vi "Calibrate_Short.vi"(8 "error in":errorcluster, 9 "Keystate":string, 10 "Stop Test":bool=TRUE, 11 "Calibration Test":bool=TRUE) -> (0 "error out":errorcluster, 5 "Calibration Short Successful":bool)   [LabVIEW 2020]
uses:
  <vilib>/Instr/_visa.llb/GPIB Status Boolean Array.ctl
  <vilib>/Utility/error.llb/DialogType.ctl
panel:
  out "ibsta":T1
  out "message":string=" INSTRUCTIONS:\r\rNormal Use:  When using subVIs that incorporate the error in/error out (or error I/O) structure, place this handler where you want to inform the user of an error, typically at the end of the I/O data path, as the last action of the program.  If the error in error? is ERROR, the handler creates a message describing the error and its source.  If the type of dialog = 1 (default), the message is displayed to the user, who can only acknowedge it.  If the type = 2, the user can acknowledge the message or abort execution; aborting a program with active I/O is not recommended.  If the type = 0, no message is displayed; this is used to process the error programmatically, and the error out cluster elements are wired to individual terminals for that reason.  \r\rOther Use:\n\r\nlocal testing.  To test the error code of a subVI or function that does not have the error I/O structure, you can wire its error code and a source string to the local error code and error source inputs.  If error in error? indicates no error and error code is not equal to 0, the local code and source are substituted for the error in values, and error? is set TRUE (ERROR)."
  out "Test Count":i32
  out "Failed Test Count":i32
  out "serial poll byte (Test 2)":i16
  out "serial poll byte (Test 1)":i16
  in  "Test Failed":bool=TRUE
  in  "Cal_Step_Delay":u16
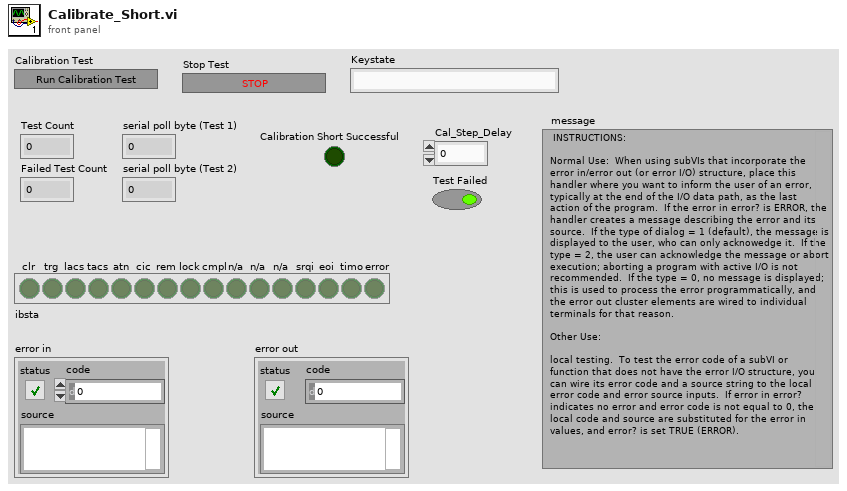
[diagram p1: front panel]
types:
  T1 = typedef "GPIB Status Boolean Array.ctl" = bool[]
  T2 = typedef "DialogType.ctl" = u16
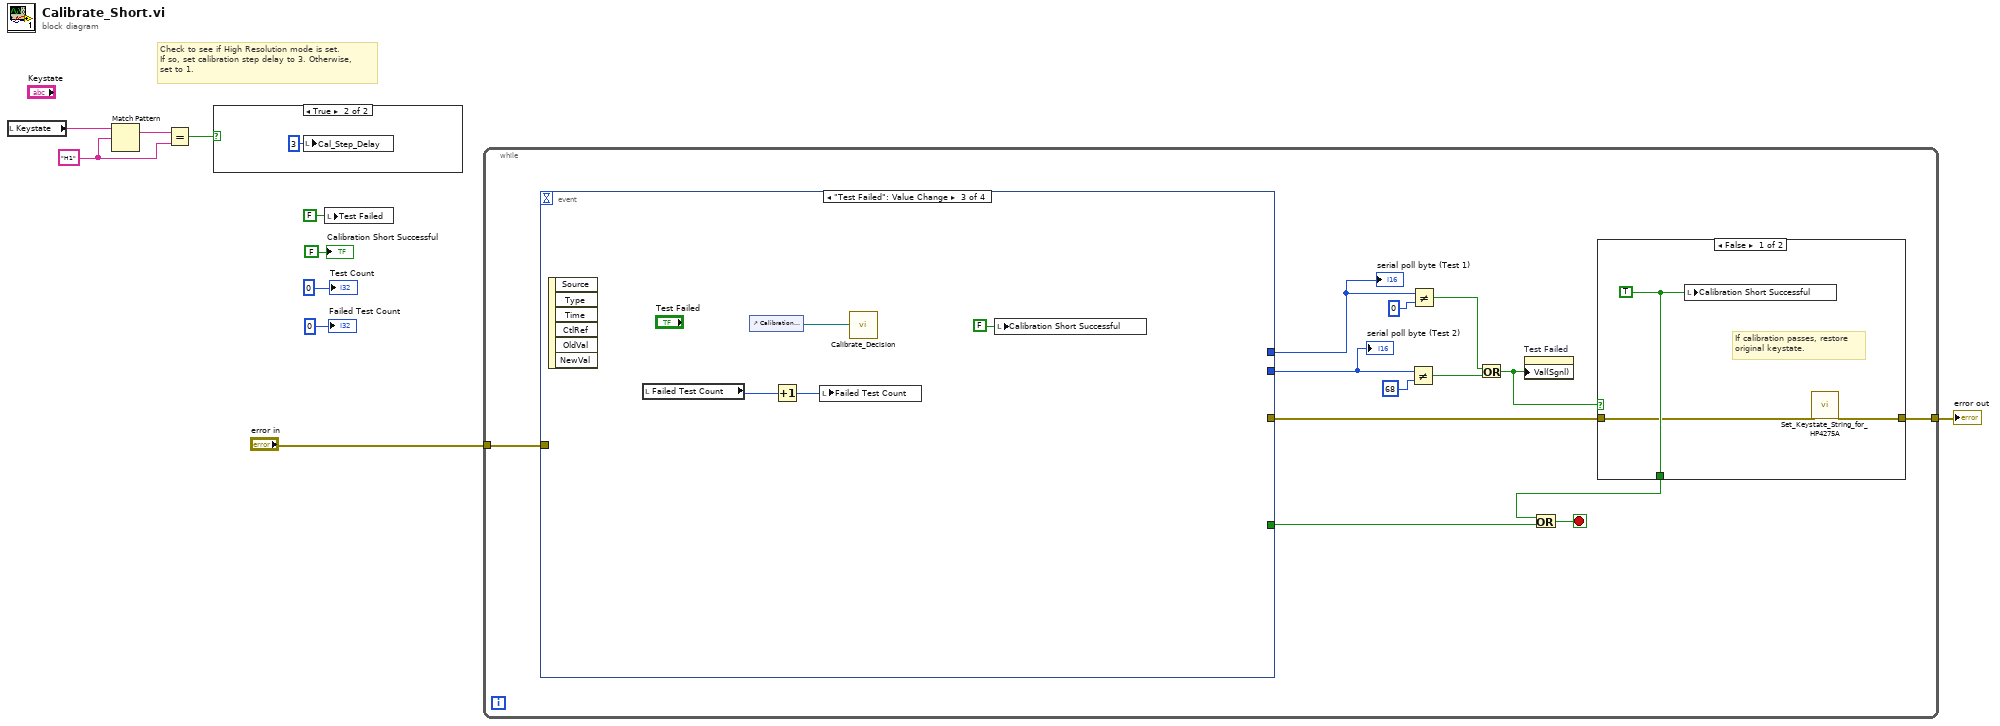
[diagram p0: block diagram]
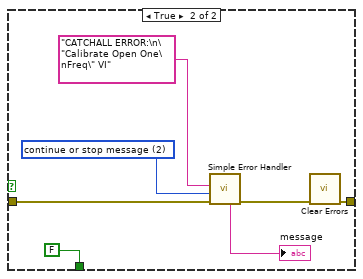
[diagram p2: hidden frame]
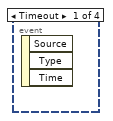
[diagram p3: hidden frame]
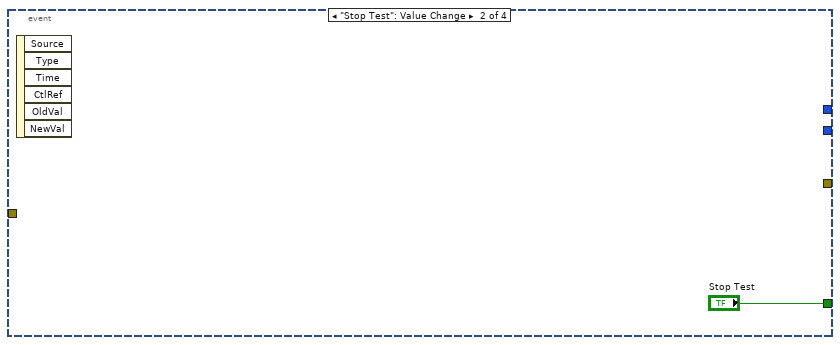
[diagram p4: hidden frame]
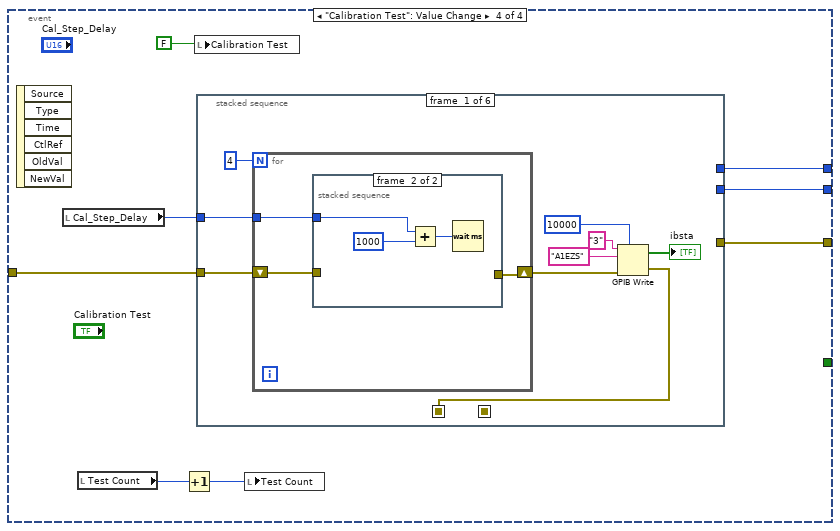
[diagram p5: hidden frame]
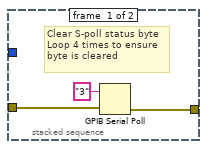
[diagram p6: hidden frame]
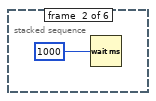
[diagram p7: hidden frame]
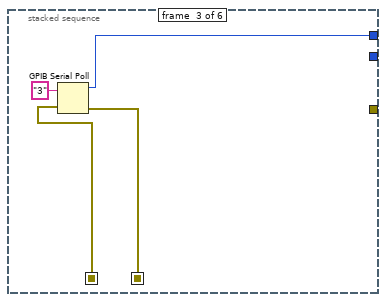
[diagram p8: hidden frame]
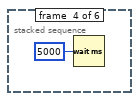
[diagram p9: hidden frame]
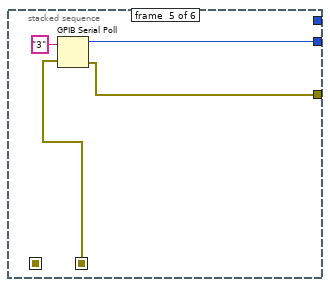
[diagram p10: hidden frame]
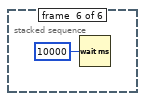
[diagram p11: hidden frame]
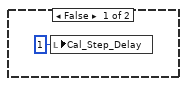
[diagram p12: hidden frame]
diagram:
  w10 = "H1" ("regular expression")
  # "Check to see if High Resolution mode is set.\nIf so, set calibration step delay to 3. Otherwise,\nset to 1."
  n1 = local read "Keystate"() -> (w6:string)
  n2 = Match Pattern(string=w6, regular expression=w10) -> (match substring=w9:string)  [unwired: 1 in, 3 out]
  n3 = Equal?(x=w9, y=w10) -> (x = y?=w8:bool)
  n4 = case shown="True" w8 {
    frame False {
      n5 = local write "Cal_Step_Delay"(u16 1 ("CalStepDelay")) -> ()
    }
    frame True {
      n6 = local write "Cal_Step_Delay"(u16 3 ("CalStepDelay")) -> ()
    }
  }
  n7 = local write "Test Failed"(FALSE ("Test Failed")) -> ()
  n8 = while {
    tunnel: "error in" -> [w25]
    tunnel: [w20] -> w7
    stop <- w22 stop-if-true
    n9 = event shown="[2] \"Test Failed\": Value Change" {
      selector: _ -> [_ _ _ _]
      dyn-events: _ -> [_ _ _ _]
      timeout: _ -> [_ _ _ _]
      tunnel: w25 -> [_ _ _ w48]
      tunnel: [_ _ _ w46] -> w21
      tunnel: [_ "Stop Test" _ _] -> w23
      tunnel: [_ _ _ w42] -> w17
      tunnel: [_ _ _ w41] -> w14
      event Timeout {
        n10 = event-data() -> ()  [unwired: 1 in, 3 out]
      }
      event "Stop Test": Value Change {
        n11 = event-data() -> ()  [unwired: 1 in, 6 out]
      }
      event "Test Failed": Value Change {
        n12 = event-data() -> ()  [unwired: 1 in, 6 out]
        n13 = local read "Failed Test Count"() -> (w40:i32)
        n14 = control-ref of="Calibration Test"() -> (w38:refnum<vi>)
        n15 = Increment(x=w40) -> (x+1=w39:i32)
        n16 = local write "Failed Test Count"(w39) -> ()
        n17 = call "Calibrate_Decision.vi"("reference"=w38) -> ()  [unwired: 11 in]
        n18 = local write "Calibration Short Successful"(FALSE ("Calibration Short Successful")) -> ()
      }
      event "Calibration Test": Value Change {
        n19 = event-data() -> ()  [unwired: 1 in, 6 out]
        n20 = local read "Cal_Step_Delay"() -> (w47:u16)
        n21 = local read "Test Count"() -> (w44:i32)
        n22 = Increment(x=w44) -> (x+1=w43:i32)
        n23 = local write "Calibration Test"(FALSE ("Calibration Test")) -> ()
        n24 = stacked-sequence {
          seq-local: [w49 _ _ _ _ _] -> [_ _ w70 _ _ _]
          seq-local: [_ _ w69 _ _ _] -> [_ _ _ _ w75 _]
          tunnel: w48 -> [w57 _ _ _ _ _]
          tunnel: w47 -> [w56 _ _ _ _ _]
          tunnel: [_ _ _ _ w74 _] -> w46
          tunnel: [_ _ w68 _ _ _] -> w42
          tunnel: [_ _ _ _ w73 _] -> w41
          frame #0 {
            n25 = for {
              N: 4 -> [_]
              tunnel: w56 -> [w59]
              shift-right: [w58] -> w50
              shift-left: w57 -> [w60]
              n26 = stacked-sequence {
                tunnel: w60 -> [w62 _]
                tunnel: w59 -> [_ w65]
                tunnel: [w61 _] -> w58
                frame #0 {
                  # "Clear S-poll status byte\nLoop 4 times to ensure\nbyte is cleared"
                  n27 = GPIB Serial Poll(0:"3" ("address string"), 1:w62) -> (4:w61:errorcluster)  [unwired: 2 out]
                }
                frame #1 {
                  n28 = Add(x=w65, y=u32 1000 ("milliseconds to wait")) -> (x+y=w64:u32)
                  n29 = Wait (ms)(milliseconds to wait=w64) -> ()  [unwired: 1 out]
                }
              }
            }
            n30 = GPIB Write(0:"3" ("address string"), 1:"A1EZS" ("data"), 3:w50, 4:10000 ("timeout ms (488.2 global)")) -> (5:→"ibsta":bool[], 6:w49:errorcluster)  [unwired: 1 in]
          }
          frame #1 {
            n31 = Wait (ms)(milliseconds to wait=u32 1000) -> ()  [unwired: 1 out]
          }
          frame #2 {
            n32 = GPIB Serial Poll(0:"3" ("address string"), 1:w70) -> (2:w68:i16, 4:w69:errorcluster)  [unwired: 1 out]
          }
          frame #3 {
            n33 = Wait (ms)(milliseconds to wait=u32 5000) -> ()  [unwired: 1 out]
          }
          frame #4 {
            n34 = GPIB Serial Poll(0:"3" ("address string"), 1:w75) -> (2:w73:i16, 4:w74:errorcluster)  [unwired: 1 out]
          }
          frame #5 {
            n35 = Wait (ms)(milliseconds to wait=u32 10000) -> ()  [unwired: 1 out]
          }
        }
        n36 = local write "Test Count"(w43) -> ()
      }
    }
    "serial poll byte (Test 1)" <- w17
    "serial poll byte (Test 2)" <- w14
    n37 = Not Equal?(x=w14, y=i16 68) -> (x != y?=w13:bool)
    n38 = Not Equal?(x=w17, y=i16 0) -> (x != y?=w16:bool)
    n39 = Or(x=w16, y=w13) -> (x .or. y?=w19:bool)
    n40 = property on="Test Failed" class="Bool (strict)"("Val(Sgnl)"=w19) -> ()  [unwired: 2 in, 2 out]
    n41 = case shown="False" w19 {
      tunnel: [w28 FALSE] -> w24
      tunnel: w21 -> [w27 w30]
      tunnel: [w26 w29] -> w20
      frame False {
        w28 = TRUE ("Calibration Short Successful")
        # "If calibration passes, restore\noriginal keystate."
        n42 = local write "Calibration Short Successful"(w28) -> ()
        n43 = call "Set_Keystate_String_for_HP4275A.vi"("error in"=w27) -> ("error out"=w26:errorcluster)  [unwired: 26 in]
      }
      frame True {
        w32 = T2 2 items=["no dialog", "OK message", "continue or stop message", "OK message + warnings", "continue/stop + warnings"] ("type of dialog (OK msg:1)")
        n44 = call <vilib>:"Simple Error Handler.vi"("error source (\" \")"="CATCHALL ERROR:\n\"Calibrate Open One\nFreq\" VI" ("error source (\" \")"), "type of dialog (OK msg:1)"=w32, "error in (no error)"=w30) -> ("error out"=w33:errorcluster, "message"=→"message":string)  [unwired: 2 in, 3 out]
        n45 = call <vilib>:"Clear Errors.vi"("error in (no error)"=w33) -> ("error out"=w29:errorcluster)  [unwired: 5 in, 1 out]
      }
    }
    n46 = Or(x=w24, y=w23) -> (x .or. y?=w22:bool)
  }
  "error out" <- w7
  "Failed Test Count" <- 0 ("Numeric")
  "Test Count" <- 0 ("Test Cout")
  "Calibration Short Successful" <- FALSE ("Calibration Short Successful")
